vi "GetDataSection.vi"(8 "error in (no error)":errorcluster caption="Error IN", 10 "SectionMap":T2, 11 "ABFFIO IN":refnum<class "ABFFIO.lvclass">) -> (0 "error out":errorcluster caption="Error OUT", 1 "DataProperties":T1, 2 "Sweep Data (3D)":sgl[][][](array[numeric]), 3 "ABFFIO OUT":refnum<class "ABFFIO.lvclass">)   [LabVIEW 2017, in "ABFFIO.lvclass"]
uses:
  ABFFIO.lvclass
  ABFFIO.lvclass/ABFFIO.ctl
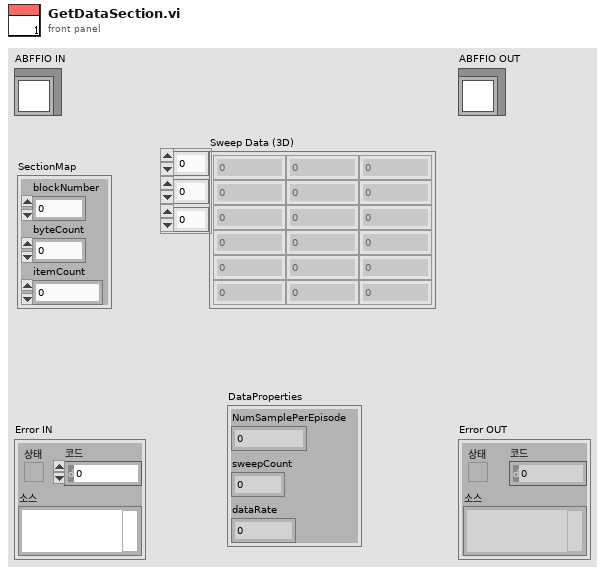
[diagram p1: front panel]
types:
  T1 = cluster{"NumSamplePerEpisode":dbl, "sweepCount":u32, "dataRate":i32}
  T2 = cluster{"blockNumber":u32, "byteCount":u32, "itemCount":u32}
  T3 = enum16{"big-endian, network order", "native, host order", "little-endian"}
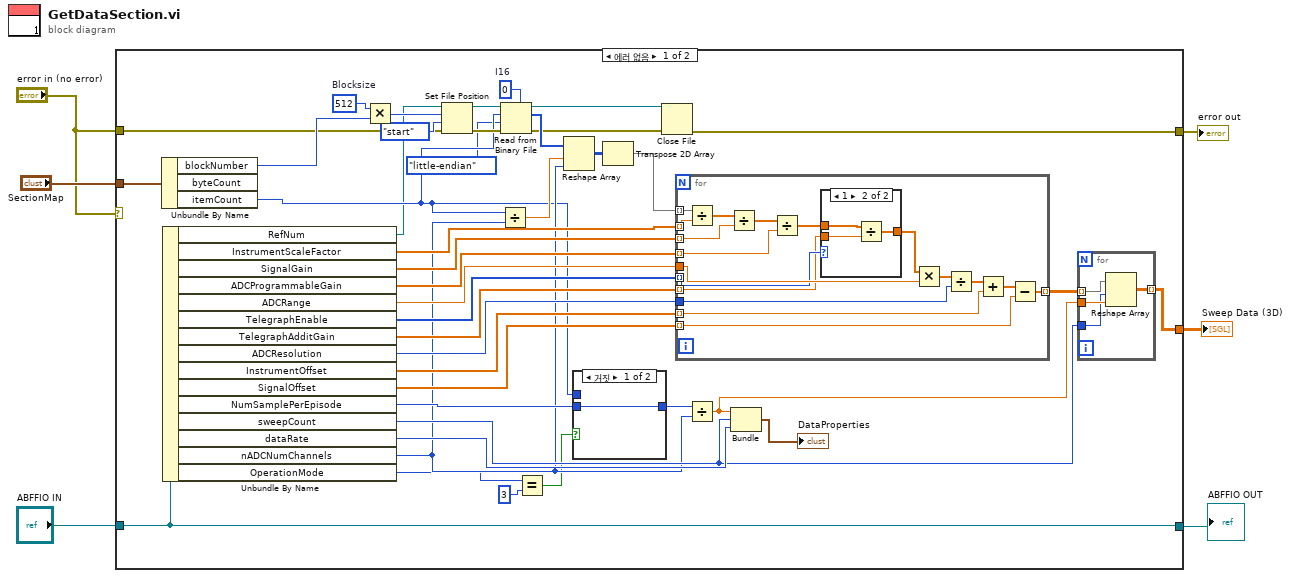
[diagram p0: block diagram]
diagram:
  n1 = case shown="에러 없음" "error in (no error)" {
    selector: "error in (no error)" -> [_ w77]
    tunnel: [w8 w77] -> w6
    tunnel: [w38 w76] -> w4
    tunnel: "ABFFIO IN" -> [w38 w76]
    tunnel: "SectionMap" -> [w47 _]
    tunnel: "error in (no error)" -> [w9 _]
    tunnel: [w7 _] -> w1
    frame No Error {
      w15 = i16 0  # I16
      w45 = u32 512  # Blocksize
      n2 = Unbundle By Name(w47) -> ("blockNumber"=w46:u32, "itemCount"=w16:u32)  [unwired: 1 out]
      n3 = Unbundle By Name(w38) -> ("RefNum"=w12:refnum<file>, "InstrumentScaleFactor"=w44:sgl[], "SignalGain"=w43:sgl[], "ADCProgrammableGain"=w42:sgl[], "ADCRange"=w41:sgl, "TelegraphEnable"=w27:u8[], "TelegraphAdditGain"=w28:sgl[], "ADCResolution"=w40:u32, "InstrumentOffset"=w39:sgl[], "SignalOffset"=w33:sgl[], "NumSamplePerEpisode"=w26:u32, "sweepCount"=w30:u32, "dataRate"=w32:i32, "nADCNumChannels"=w24:u32, "OperationMode"=w23:u8)
      n4 = Multiply(x=w45, y=w46) -> (x*y=w17:u32)
      n5 = Set File Position(offset (in bytes) (0)=w17, refnum=w12, from (0:start)=enum16{"start", "end", "current"}."start", error in=w9) -> (refnum out=w20:refnum<file>, error out=w18:errorcluster)
      n6 = Divide(x=w16, y=w24) -> (x/y=w36:dbl)
      n7 = Read from Binary File(5:w15, 8:w18, 9:T3."little-endian" ("byte order (0:big-endian, network order)"), 10:w16, 11:w20) -> (0:w11:errorcluster, 2:w13:i16[], 3:w10:refnum<file>)  [unwired: 1 in, 1 out]
      n8 = Equal?(x=w23, y=u8 3) -> (x = y?=w21:bool)
      n9 = Reshape Array(w13, w36, w24) -> (w35:i16[][])
      n10 = case shown="거짓" w21 {
        tunnel: w26 -> [w48 _]
        tunnel: [w48 w49] -> w25
        tunnel: w16 -> [_ w49]
        frame False {
        }
        frame True {
        }
      }
      n11 = Transpose 2D Array(2D array=w35) -> (transposed array=w34:i16[][])
      n12 = Close File(refnum=w10, error in=w11) -> (error out=w8:errorcluster)  [unwired: 1 out]
      n13 = for {
        tunnel: w44 -> [w71] mode=indexing
        tunnel: w43 -> [w69] mode=indexing
        tunnel: w42 -> [w68] mode=indexing
        tunnel: w41 -> [w66]
        tunnel: w40 -> [w64]
        tunnel: w39 -> [w62] mode=indexing
        tunnel: w34 -> [w61] mode=indexing
        tunnel: [w59] -> w31 mode=indexing
        tunnel: w33 -> [w58] mode=indexing
        tunnel: w28 -> [w54] mode=indexing
        tunnel: w27 -> [w57] mode=indexing
        n14 = Divide(x=w61, y=w71) -> (x/y=w70:sgl[])
        n15 = Divide(x=w70, y=w69) -> (x/y=w67:sgl[])
        n16 = Divide(x=w67, y=w68) -> (x/y=w56:sgl[])
        n17 = case shown="1" w57 {
          tunnel: w56 -> [w72 w75]
          tunnel: [w72 w73] -> w55
          tunnel: w54 -> [_ w74]
          frame 0, Default {
          }
          frame 1 {
            n18 = Divide(x=w75, y=w74) -> (x/y=w73:sgl[])
          }
        }
        n19 = Multiply(x=w55, y=w66) -> (x*y=w65:sgl[])
        n20 = Divide(x=w65, y=w64) -> (x/y=w63:sgl[])
        n21 = Add(x=w63, y=w62) -> (x+y=w60:sgl[])
        n22 = Subtract(x=w60, y=w58) -> (x-y=w59:sgl[])
      }
      n23 = Divide(x=w25, y=w24) -> (x/y=w29:dbl)
      n24 = Bundle(w29, "sweepCount"=w30, "dataRate"=w32) -> (→"DataProperties":cluster{dbl, "sweepCount":u32, "dataRate":i32})  [unwired: 1 in]
      n25 = for {
        tunnel: w31 -> [w53] mode=indexing
        tunnel: w30 -> [w50]
        tunnel: w29 -> [w51]
        tunnel: [w52] -> w7 mode=indexing
        n26 = Reshape Array(w53, w50, w51) -> (w52:sgl[][])
      }
    }
    frame Error {
    }
  }
  "error out" <- w6
  "ABFFIO OUT" <- w4
  "Sweep Data (3D)" <- w1
